vi "Measurements.vi"() -> ()   [LabVIEW 2015]
uses:
  <vilib>/Analysis/Matrix/Numeric/Conversions/Array To Matrix - RA.vi
  <vilib>/express/express arith-compare/Formula/XNode/ExpressFormulaBlockNode.xnode
  <vilib>/Analysis/NI_AALPro.lvlib
  <vilib>/Analysis/Matrix/NI_Matrix.lvlib
panel:
  in  "Wire sample diameter, um (metal core only)":dbl=10.0
  in  "VISA Generator":refnum<visa-resource-name>="Generator"
  in  "Write to the file":bool
  in  "Ground level noise amplitude (trigger level), V":dbl
  in  "Voltage to Gauss coefficient , V*s/(G*rad*m^2)":dbl=1.2
  out "Helmholtz coil current amplitude, A":dbl(knob) scale=0.0..3.0
  in  "Generator voltage , V (control the current below)":dbl=1.0
  out "BH loop":cluster{"Array":dbl[], "Array 2":dbl[]}(graph)
  in  "BH-loop (choose a name ***.csv)":path=path "C:/Users/ZJUcomposite/Desktop/Other algorithms/BH-loop/BHloop.csv"
  in  "Current to field coefficient, Oe/A":dbl=21.06
  in  "Ground level BP-filter width, Hz (5 Hz defaultt)":dbl=5.0 format="%#_13g"
  in  "BH-loop averages (20 default)":i32=20
  in  "Number of missed periods (3-5 recommended)":i32=5
  out "Waveform before integration":cluster{"Array":dbl[], "Array 2":dbl[]}(graph)
  in  "Cluster":cluster{"Array":dbl[], "Array 2":dbl[]}
  in  "Coil\namplitude\nbalance":dbl(slide) scale=-2.5..2.5
  in  "Sampling rate, Hz (100 kHz default)":dbl=100000.0 format="%#_13g"
  in  "Generator frequency, Hz":dbl=85.0 format="%#_13g"
  in  "Noise filter ratio (0.9 default)":dbl=0.9 format="%#_13g"
  in  "Noise high cutoff (<20 kHz), Hz":dbl=10000.0 format="%#_13g"
  # "Yujie Zhao & Dmitriy Makhnovskiy\nJune 2019, Hangzhou, China."
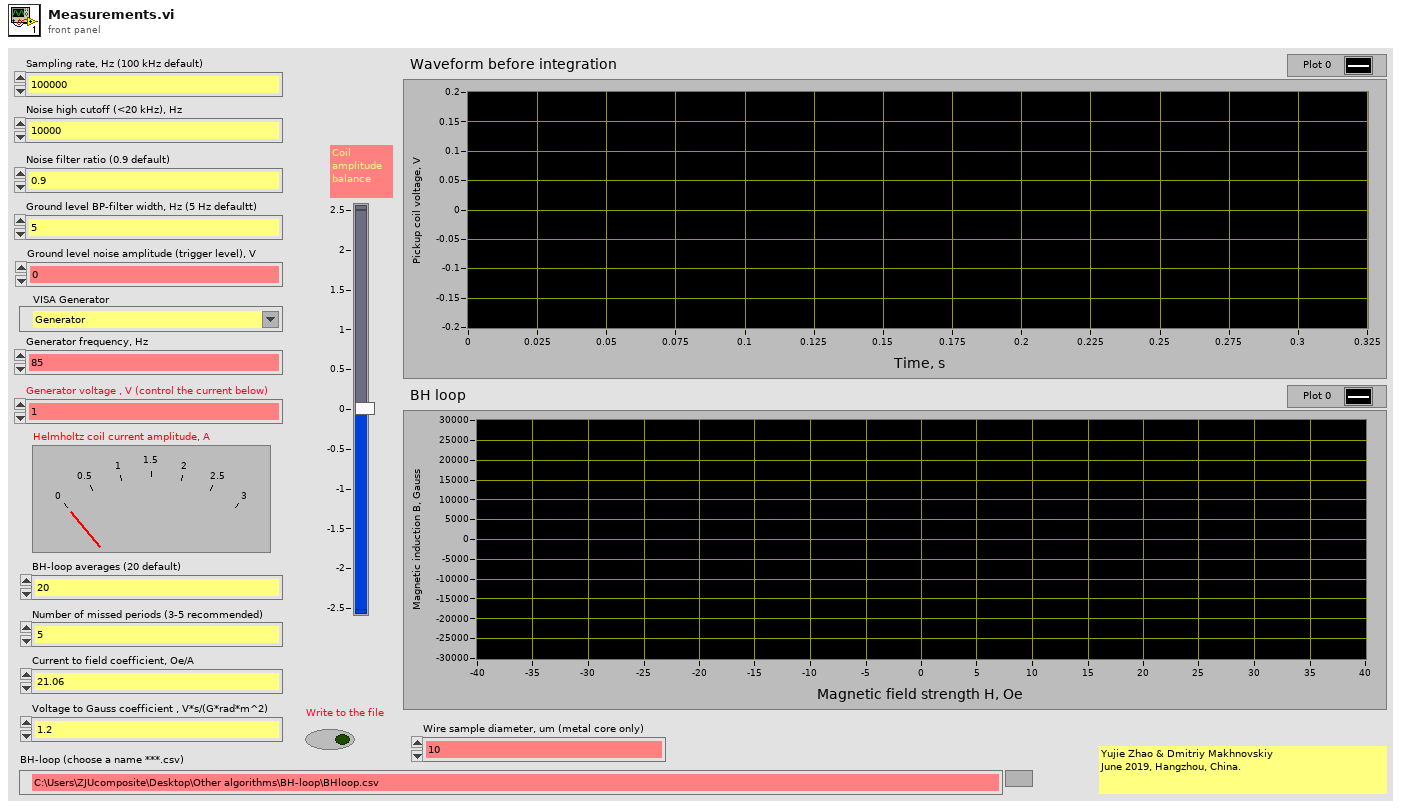
[diagram p1: front panel]
types:
  T1 = typedef "NI_Matrix.lvlib/RealMatrix.ctl" = dbl[][]
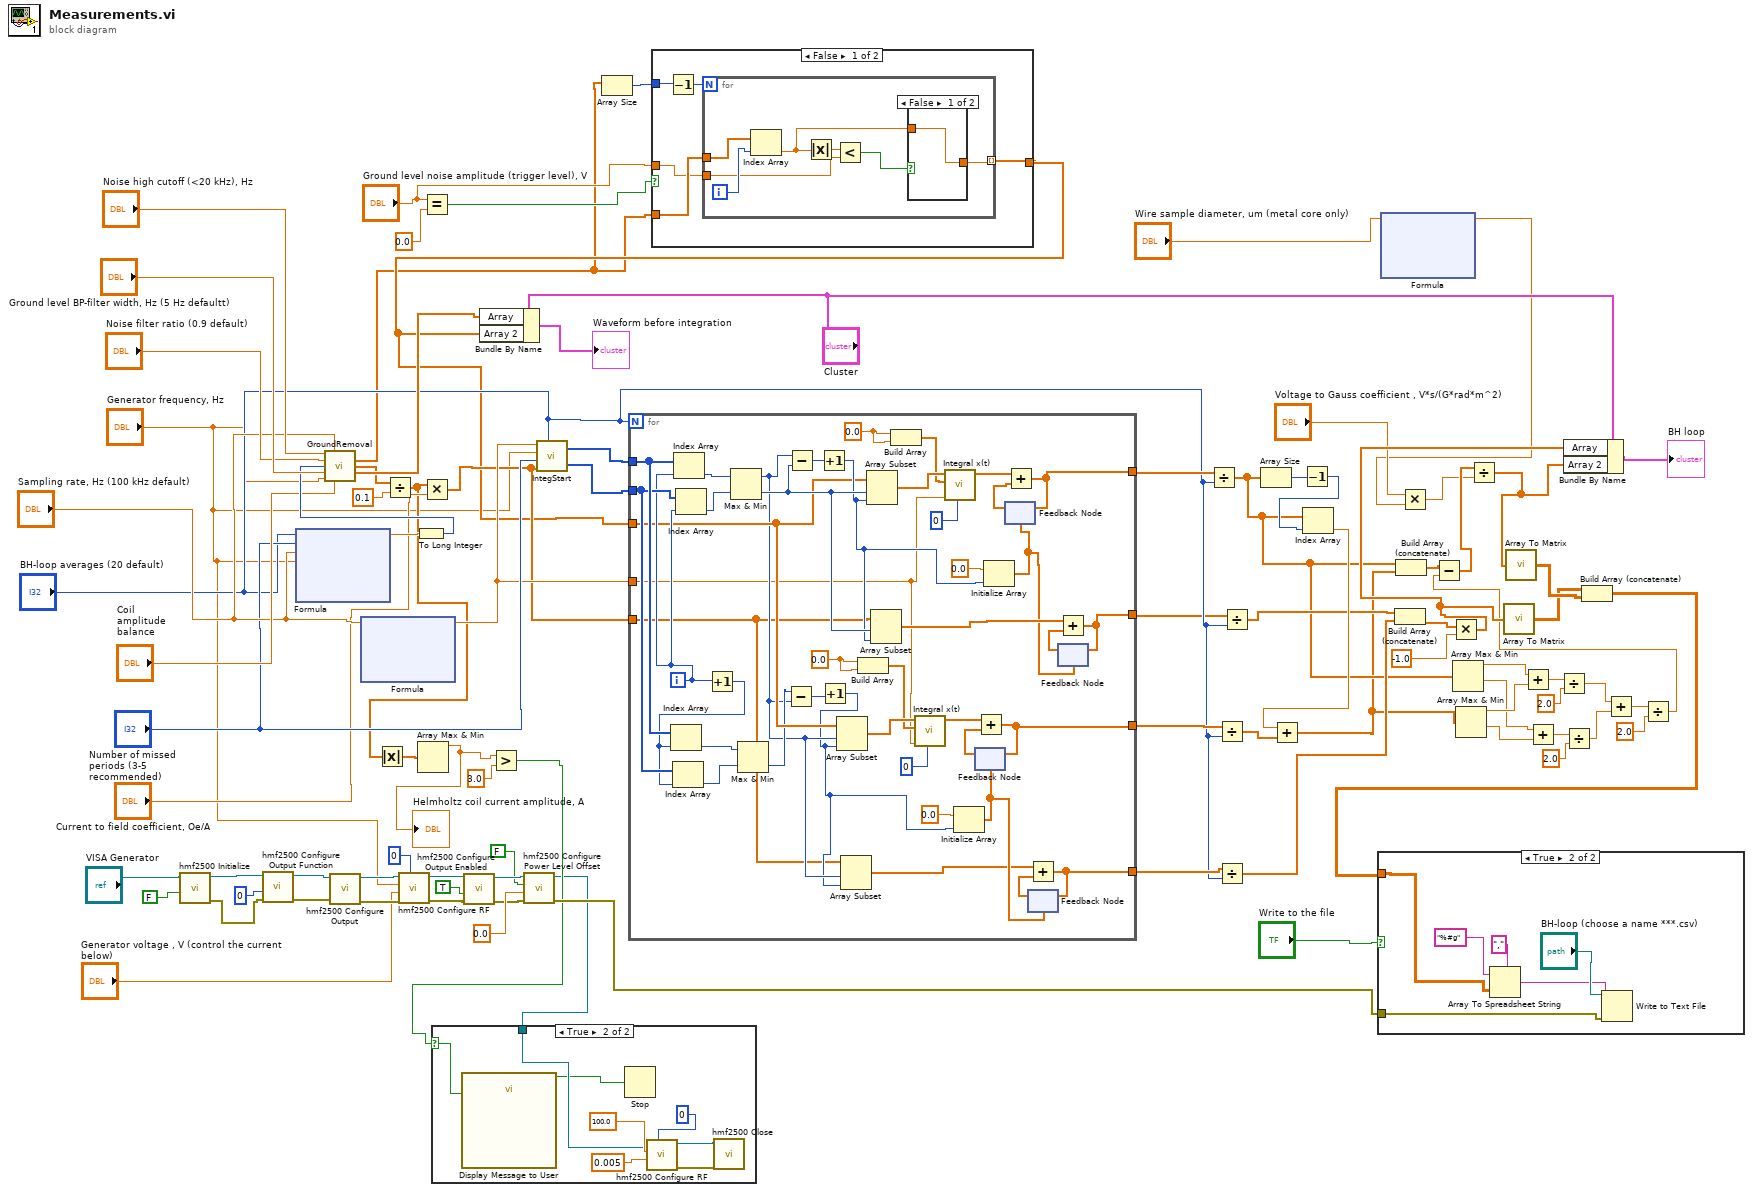
[diagram p0: block diagram]
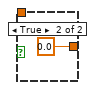
[diagram p4: hidden frame]
diagram:
  n1 = call <instrlib>:"hmf2500 Initialize.vi"("Reset (Reset)"=FALSE, "VISA resource name"="VISA Generator") -> ("error out"=w25:errorcluster, "VISA resource name out"=w27:refnum<visa-resource-name>)  [unwired: 8 in]
  n2 = call <instrlib>:"hmf2500 Configure Output Function.vi"("error in (no error)"=w25, "Output Function (Sinus)"=0, "VISA resource name"=w27) -> ("error out"=w23:errorcluster, "VISA resource name out"=w24:refnum<visa-resource-name>)  [unwired: 7 in]
  n3 = xnode "Formula"("N1"="BH-loop averages (20 default)", "N2"="Number of missed periods (3-5 recommended)", "fs"="Sampling rate, Hz (100 kHz default)", "fg"="Generator frequency, Hz") -> ("Result"=w87:dbl)  [unwired: 1 in, 1 out]
  n4 = call <instrlib>:"hmf2500 Configure Output.vi"("error in (no error)"=w23, "VISA resource name"=w24) -> ("error out"=w21:errorcluster, "VISA resource name out"=w22:refnum<visa-resource-name>)  [unwired: 8 in]
  n5 = xnode "Formula"("fs"="Sampling rate, Hz (100 kHz default)") -> ("Result"=w79:dbl)  [unwired: 1 in, 1 out]
  n6 = call <instrlib>:"hmf2500 Configure RF.vi"("Amplitude Unit (Volt)"=0, "error in (no error)"=w21, "Power Level (0.2)"="Generator voltage , V (control the current below)", "Frequency (1.0E6)"="Generator frequency, Hz", "VISA resource name"=w22) -> ("error out"=w16:errorcluster, "VISA resource name out"=w17:refnum<visa-resource-name>)  [unwired: 5 in]
  n7 = To Long Integer(number=w87) -> (32bit integer=w86:i32)
  n8 = call "GroundRemoval.vi"("Noise high cutoff, Hz"="Noise high cutoff (<20 kHz), Hz", "Sampling rate, Hz"="Sampling rate, Hz (100 kHz default)", "Noise filter ratio"="Noise filter ratio (0.9 default)", "Number of samplings"=w86, "Ground level BP-filter width, Hz"="Ground level BP-filter width, Hz (5 Hz defaultt)", "Generator frequency, Hz"="Generator frequency, Hz", "Slide"="Coil\namplitude\nbalance") -> ("Final Waveform"=w33:dbl[], "Field"=w42:dbl[], "Time"=w80:dbl[])  [unwired: 5 in, 1 out]
  n9 = Divide(x=w42, y=0.1) -> (x/y=w40:dbl[])
  n10 = Absolute Value(x=w40) -> (abs(x)=w39:dbl[])
  n11 = Array Max & Min(array=w39) -> (max value=w7:dbl)  [unwired: 3 out]
  "Helmholtz coil current amplitude, A" <- w7
  n12 = Equal?(x="Ground level noise amplitude (trigger level), V", y=0.0) -> (x = y?=w37:bool)
  n13 = Multiply(x=w40, y="Current to field coefficient, Oe/A") -> (x*y=w41:dbl[])
  n14 = call <instrlib>:"hmf2500 Configure Output Enabled.vi"("error in (no error)"=w16, "Output Enabled (On)"=TRUE, "VISA resource name"=w17) -> ("error out"=w11:errorcluster, "VISA resource name out"=w14:refnum<visa-resource-name>)  [unwired: 7 in]
  n15 = Greater?(x=w7, y=3.0) -> (0:w8:bool)
  n16 = call <instrlib>:"hmf2500 Configure Power Level Offset.vi"("error in (no error)"=w11, "Power Level Offset (5.0)"=0.0, "Power Level (Off)"=FALSE, "VISA resource name"=w14) -> ("error out"=w10:errorcluster, "VISA resource name out"=w1:refnum<visa-resource-name>)  [unwired: 6 in]
  n17 = case shown="True" w8 {
    selector: w8 -> [_ w93]
    tunnel: w1 -> [_ w94]
    frame False {
    }
    frame True {
      n18 = call "Display Message to User"("Enable"=w93) -> ("OK"=w92:bool)  [unwired: 9 in, 1 out]
      n19 = Stop(stop? (T)=w92) -> ()
      n20 = call <instrlib>:"hmf2500 Configure RF.vi"("Amplitude Unit (Volt)"=0, "Power Level (0.2)"=0.005, "Frequency (1.0E6)"=100.0, "VISA resource name"=w94) -> ("error out"=w96:errorcluster, "VISA resource name out"=w95:refnum<visa-resource-name>)  [unwired: 6 in]
      n21 = call <instrlib>:"hmf2500 Close.vi"("error in (no error)"=w96, "VISA resource name"=w95) -> ()  [unwired: 9 in, 1 out]
    }
  }
  n22 = call "IntegStart.vi"("Time step"=w79, "Generator frequency"="Generator frequency, Hz", "Number of ignored periods"="Number of missed periods (3-5 recommended)", "Field"=w41, "BH averages"="BH-loop averages (20 default)") -> ("Min Index"=w82:i32[], "Max Index"=w81:i32[])
  n23 = Array Size(array=w33) -> (size(s)=w34:i32)
  n24 = case shown="False" w37 {
    tunnel: w33 -> [w104 w114]
    tunnel: [w100 w114] -> w36
    tunnel: "Ground level noise amplitude (trigger level), V" -> [w101 _]
    tunnel: w34 -> [w102 _]
    frame False {
      n25 = Decrement(x=w102) -> (x-1=w103:i32)
      n26 = for {
        N: w103 -> [_]
        tunnel: w104 -> [w110]
        tunnel: w101 -> [w109]
        tunnel: [w108] -> w100 mode=indexing
        i -> [w111]
        n27 = Index Array(array=w110, index=w111) -> (element=w106:dbl)
        n28 = Absolute Value(x=w106) -> (abs(x)=w105:dbl)
        n29 = Less?(x=w105, y=w109) -> (x < y?=w107:bool)
        n30 = case shown="False" w107 {
          tunnel: [w112 0.0] -> w108
          tunnel: w106 -> [w112 _]
          frame False {
          }
          frame True {
          }
        }
      }
    }
    frame True {
    }
  }
  n31 = Bundle By Name(cluster="Cluster", "Array"=w80, "Array 2"=w36) -> (→"Waveform before integration":cluster{"Array":dbl[], "Array 2":dbl[]})
  n32 = for {
    N: "BH-loop averages (20 default)" -> [_]
    tunnel: w82 -> [w139]
    tunnel: w81 -> [w138]
    tunnel: w36 -> [w124]
    tunnel: w79 -> [w115]
    tunnel: [w148] -> w78
    tunnel: w41 -> [w118]
    tunnel: [w140] -> w74
    tunnel: [w123] -> w77
    tunnel: [w116] -> w76
    i -> [w137]
    w132 = 0.0
    w153 = 0.0
    n33 = Index Array(array=w139, index=w137) -> (element=w155:i32)
    n34 = Index Array(array=w138, index=w137) -> (element=w156:i32)
    n35 = Increment(x=w137) -> (x+1=w136:i32)
    n36 = Index Array(array=w139, index=w136) -> (element=w135:i32)
    n37 = Index Array(array=w138, index=w136) -> (element=w134:i32)
    n38 = Max & Min(x=w155, y=w156) -> (max(x,y)=w120:i32, min(x,y)=w145:i32)
    n39 = Max & Min(x=w135, y=w134) -> (min(x,y)=w121:i32)  [unwired: 1 out]
    n40 = Subtract(x=w121, y=w120) -> (x-y=w122:i32)
    n41 = Subtract(x=w120, y=w145) -> (x-y=w150:i32)
    n42 = Increment(x=w150) -> (x+1=w144:i32)
    n43 = Increment(x=w122) -> (x+1=w119:i32)
    n44 = Array Subset(array=w124, index=w120, length=w119) -> (w133:dbl[])
    n45 = Array Subset(array=w118, index=w120, length=w119) -> (w117:dbl[])
    n46 = Build Array(w132, w132) -> (w131:dbl[])
    n47 = Array Subset(array=w124, index=w145, length=w144) -> (w154:dbl[])
    n48 = Array Subset(array=w118, index=w145, length=w144) -> (w143:dbl[])
    n49 = Build Array(w153, w153) -> (w152:dbl[])
    n50 = call <vilib>:"Integral x(t).vi"("integration method"=0, "dt"=w115, "Initial Condition"=w131, "X"=w133) -> ("Integral X"=w127:dbl[])  [unwired: 6 in, 1 out]
    n51 = call <vilib>:"Integral x(t).vi"("integration method"=0, "dt"=w115, "Initial Condition"=w152, "X"=w154) -> ("Integral X"=w146:dbl[])  [unwired: 6 in, 1 out]
    n52 = Initialize Array(0.0, w119) -> (w125:dbl[])
    n53 = feedback #1(w125) -> (w129:dbl[])
    n54 = Add(x=w127, y=w129) -> (x+y=w123:dbl[])
    n55 = feedback-in #1(w123) -> ()
    n56 = Initialize Array(0.0, w144) -> (w141:dbl[])
    n57 = feedback #2(w141) -> (w149:dbl[])
    n58 = Add(x=w146, y=w149) -> (x+y=w148:dbl[])
    n59 = feedback-in #2(w148) -> ()
    n60 = feedback #3(w125) -> (w126:dbl[])
    n61 = Add(x=w117, y=w126) -> (x+y=w116:dbl[])
    n62 = feedback-in #3(w116) -> ()
    n63 = feedback #4(w141) -> (w142:dbl[])
    n64 = Add(x=w143, y=w142) -> (x+y=w140:dbl[])
    n65 = feedback-in #4(w140) -> ()
  }
  n66 = Divide(x=w78, y="BH-loop averages (20 default)") -> (x/y=w60:dbl[])
  n67 = Divide(x=w77, y="BH-loop averages (20 default)") -> (x/y=w70:dbl[])
  n68 = Divide(x=w76, y="BH-loop averages (20 default)") -> (x/y=w68:dbl[])
  n69 = Divide(x=w74, y="BH-loop averages (20 default)") -> (x/y=w69:dbl[])
  n70 = Array Size(array=w60) -> (size(s)=w73:i32)
  n71 = Decrement(x=w73) -> (x-1=w72:i32)
  n72 = Index Array(array=w60, index=w72) -> (element=w71:dbl)
  n73 = Add(x=w71, y=w70) -> (x+y=w59:dbl[])
  n74 = xnode "Formula"("X1"="Wire sample diameter, um (metal core only)") -> ("Result"=w3:dbl)  [unwired: 1 in, 1 out]
  n75 = Build Array (concatenate)(w69, w68) -> (w63:dbl[])
  n76 = Build Array (concatenate)(w60, w59) -> (w46:dbl[])
  n77 = Multiply(x="Voltage to Gauss coefficient , V*s/(G*rad*m^2)", y=w3) -> (x*y=w2:dbl)
  n78 = Multiply(x=w63, y=-1.0) -> (x*y=w61:dbl[])
  n79 = Array Max & Min(array=w60) -> (max value=w58:dbl, min value=w52:dbl)  [unwired: 2 out]
  n80 = Array Max & Min(array=w59) -> (max value=w57:dbl, min value=w51:dbl)  [unwired: 2 out]
  n81 = call-poly <vilib>:"Array To Matrix.vi"("Real 1D Array"=w61) -> ("Real Matrix (Column Vector)"=w66:T1)
  n82 = Add(x=w58, y=w57) -> (x+y=w56:dbl)
  n83 = Add(x=w52, y=w51) -> (x+y=w54:dbl)
  n84 = Divide(x=w56, y=2.0) -> (x/y=w50:dbl)
  n85 = Divide(x=w54, y=2.0) -> (x/y=w49:dbl)
  n86 = Add(x=w50, y=w49) -> (x+y=w48:dbl)
  n87 = Divide(x=w48, y=2.0) -> (x/y=w45:dbl)
  n88 = Subtract(x=w46, y=w45) -> (x-y=w5:dbl[])
  n89 = Divide(x=w5, y=w2) -> (x/y=w4:dbl[])
  n90 = call-poly <vilib>:"Array To Matrix.vi"("Real 1D Array"=w4) -> ("Real Matrix (Column Vector)"=w67:T1)
  n91 = Bundle By Name(cluster="Cluster", "Array"=w61, "Array 2"=w4) -> (→"BH loop":cluster{"Array":dbl[], "Array 2":dbl[]})
  n92 = Build Array (concatenate)(w66, w67) -> (w30:T1)
  n93 = case shown="True" "Write to the file" {
    tunnel: w30 -> [_ w158]
    tunnel: w10 -> [_ w157]
    frame False {
    }
    frame True {
      n94 = Array To Spreadsheet String(delimiter (Tab)=",", array=w158, 3:"%#g") -> (spreadsheet string=w159:string)
      n95 = Write to Text File(file (use dialog)="BH-loop (choose a name ***.csv)", text=w159, error in=w157) -> ()  [unwired: 1 in, 3 out]
    }
  }
